vi "devices.vi"(8 "error in (no error)":errorcluster, 11 "reference in":refnum<class "Project Panels.lvclass">=refnum) -> (0 "error out":errorcluster, 3 "reference out":refnum<class "Project Panels.lvclass">)   [LabVIEW 2015, in "Project Panels.lvclass"]
uses:
  Project Panels.lvclass
  state.ctl
  <vilib>/Utility/miscctls.llb/LVRowAndColumnUnsignedTypeDef.ctl
  SYS/Devices Controller_llb/deviceType.ctl
  <vilib>/Utility/miscctls.llb/LVRowAndColumnTypeDef.ctl
  APP/excelFile_class/fileType.ctl
  SYS/Devices Controller_llb/Devices Controller.lvclass
  SYS/File Controller_llb/File Controller.lvclass
  APP/excelFile_class/excelFile.lvclass
panel:
  out "title":string="Cosmed Asia Pacific - Products in Aussie"
  in  "tables":T1(tab)
  out "K5":string[][](table)=[["705001", "not active", "K4b2", "not active", "not active", "not active", "not active", "not active", "not active", "not active", "not active", "not active", ""], ["803033", "not active", "K4b2", "not active", "not active", "not active", "not active", "not active", "not active", "not active", "not active", "not active", ""], ["804042", "not active", "K4b2", "not active", "not active", "not active", "not active", "not active", "not active", "not active", "not active", "not active", ""], ["804046", "", "K4b2", "Univ. of Queensland", "St Lucia, Brisbane", "Gary Wilson", "seant@hms.uq.edu.au", "Bellamby", "sep-06", "Italy", "sep-07", "not active", ""], ["804047", "not active", "K4b2", "not active", "not active", "not active", "not active", "not active", "not active", "not active", "not active", "not active", ""], ["9806059", "6.2", "K4b2", "not active", "not active", "not active", "not active", "not active", "not active", "not active", "not active", "not active", ""], ["9806062", "5.1", "K4b2", "Queensland Academy of Sport", "Sunnybank", "Mark Andrews", "mark.andrews@srq.qld.com.au", "Nahtan, GC", "june 2013 in italy for CO2 refurbish", "Italy service", "jun-14", "", ""], ["9807077", "6.0a", "K4b2", "Uni of Canterbury", "Uni of Canterbury", "Gavin Blackwell", "gavin.blackwell@canterbury.ac.nz", "Christchurch", "feb-13", "fede", "feb-14", "", ""], ["9810080", "", "K4b2", "Royal Children's Hospital", "Herston", "Teresa Phillips", "Teresa_Phillips@health.qld.gov.au", "Herston", "jun-06", "Italy", "jun-07", "9/17/2013", ""], ["9903123", "7.2", "K4b2", "Uni of Adelaide", "Uni of Adelaide", "David Bentley", "david.bentley@adelaide.edu.au", "Adelaide", "dic-12", "Serv Italy +valve", "dic-13", "", ""], ["9912206", "7.3", "K4b2", "Uni of Canterbury", "Uni of Canterbury", "Gavin Blackwell", "gavin.blackwell@canterbury.ac.nz", "Christchurch", "feb-13", "fede", "feb-14", "", ""], ["200104325", "8", "K4b2", "Uni of South Australia", "Sansom Institute", "Michelle N. McDonnell", "", "Adelaide", "nov-11", "fede", "dic-12", "9/9/2013", ""], ["200201385", "9.1b", "K4b2", "University of Sydney", "Lidcombe Campus", "Hui Yin Ler  (PhD)", "", "Sydney", "oct-11", "fede", "oct-12", "9/9/2013", ""], ["200205419", "8.0", "K4b2", "University of Sydney", "Liverpool hospital", "Leanne Hassett", "leanne.hassett@sydney.edu.au", "Sydney", "nov-11", "fede", "nov-12", "Not Using in this moment", ""], ["200205423", "9.1b", "K4b2", "University of Sydney", "Lidcombe Campus", "Martin Thomson", "", "Sydney", "feb-10", "italy", "feb-11", "9/9/2013", ""], ["200205424", "7.3", "K4b2", "University of Sydney", "Lidcombe Campus", "Martin Thomson", "", "Sydney", "sep-08", "Italy", "sep-09", "9/10/2013", ""], ["200404607", "", "K4b2", "The Sydney Children's Hospital Network", "Westmead", "Leanne Purcell", "leanne.purcell@health.nsw.gov.au", "Westmead", "nov-08", "italy", "nov-09", "9/17/2013", "Yes, but waiting the start of the testing"], ["200512701", "8.0b", "K4b2", "James Cook Uni", "James Cook Uni", "Anthony Leight", "Anthony.Leicht@jcu.edu.au", "Townsville", "jan-13", "", "jan-14", "", ""], ["200601705", "", "K4b2", "Latrobe University", "Bundoora (Melb)", "Paul Moon", "P.Moon@latrobe.edu.au", "Melbourne", "jan-08", "Italy", "jan-09", "9/17/2013", ""], ["200607745", "", "K4b2", "QUT Brisbane", "Kelvin Grove", "Pei Cher", "pei.cher@qut.edu.au", "BBN", "may-13", "fede", "may-14", "", ""], ["200710813", "", "K4b2", "Victoria Uni", "", "Jessica Meilak", "jessica.meilak@vu.edu.au", "Melb", "jan-12", "Brad", "jan-14", "15/01/14", ""], ["200907909", "9.1b", "K4b2", "Uni of New South Wales", "Uni of New South Wales", "Stephen Redmond", "s.redmond@unsw.edu.au", "Sydney", "sep-12", "fede", "sep-13", "9/17/2013", ""], ["200909916", "", "K4b2", "Uni of Canterbury", "Uni of Canterbury", "Gavin Blackwell", "gavin.blackwell@canterbury.ac.nz", "Christchurch", "feb-13", "fede", "feb-14", "", ""], ["201007964", "", "K4b2", "University of Canberra", "Canberra", "Ben Rattray", "ben.rattray@canberra.edu.au", "Canberra", "mar-12", "", "mar-13", "9/17/2013", ""], ["201009980", "9.1b", "K4b2", "Uni of Technology Sydney", "UTS City Campus", "Steven Su", "steven.su@eng.uts.edu.au", "Sydney", "oct-12", "Medtel (also Lee Valve)", "oct-13", "9/17/2013", ""], ["2011121063", "", "K4b2", "Victoria Uni", "", "Jessica Meilak", "jessica.meilak@vu.edu.au", "Melb", "jan-12", "Brad", "jan-14", "", ""], ["2011121064", "", "K4b2", "Victoria Uni", "", "Jessica Meilak", "jessica.meilak@vu.edu.au", "Melb", "jan-12", "Brad", "jan-14", "", ""], ["2012021076", "", "K4b2", "Demo Unit", "Demo Unit", "TBD", "", "TBD", "sep-13", "Manu-AUS", "sep-14", "", ""], ["2012021080", "", "K4b2", "Massey Univ.", "Wellington", "Brandon Woolley", "B.Woolley@massey.ac.nz", "Wellington", "nov-13", "Manu-AUS", "nov-14", "", ""], ["2012061109", "", "K4b2", "Griffith University Gold Coast Campus", "Gold Coast", "Anna Boehm", "a.boehm@griffith.edu.au", "Gold Coast", "jul-13", "fede", "jul-14", "", ""], ["2012061115", "10.0d", "K4b2", "University of Newcastle", "Callaghan", "Robin Callister", "Robin.Callister@newcastle.edu.au", "Ourimbah", "nov-13", "Manu-AUS", "nov-14", "", ""], ["2012111144", "10.0d", "K4b2", "University of Newcastle", "Callaghan", "Robin Callister", "Robin.Callister@newcastle.edu.au", "Ourimbah", "nov-13", "Manu-AUS", "nov-14", "", ""], ["2012111148", "", "K4b2", "University of Western Sydney", "PENRITH", "Tara Hamilton", "t.hamilton@uws.edu.au", "PENRITH", "dec-13", "Manu-AUS", "dec-14", "", ""], ["2013011158", "10.0d", "K4b2", "University of the Sunshine Coast", "Maroochydore DC", "Ava Kerr", "akerr@usc.edu.au", "Sippy Downs", "may-13", "new", "may-14", "", ""], ["2013031168", "10.0d", "K4b2", "Australian Catholic University", "Sydney", "Phillip Chapman", "Phillip.Chapman@acu.edu.au", "Sydney", "apr-13", "new", "apr-14", "", ""], ["Prova", "", "Prova", "", "", "", "", "", "", "", "", "", ""]]
  out "k4b2":string[][](table)=[["705001", "not active", "K4b2", "not active", "not active", "not active", "not active", "not active", "not active", "not active", "not active", "not active", ""], ["803033", "not active", "K4b2", "not active", "not active", "not active", "not active", "not active", "not active", "not active", "not active", "not active", ""], ["804042", "not active", "K4b2", "not active", "not active", "not active", "not active", "not active", "not active", "not active", "not active", "not active", ""], ["804046", "", "K4b2", "Univ. of Queensland", "St Lucia, Brisbane", "Gary Wilson", "seant@hms.uq.edu.au", "Bellamby", "sep-06", "Italy", "sep-07", "not active", ""], ["804047", "not active", "K4b2", "not active", "not active", "not active", "not active", "not active", "not active", "not active", "not active", "not active", ""], ["9806059", "6.2", "K4b2", "not active", "not active", "not active", "not active", "not active", "not active", "not active", "not active", "not active", ""], ["9806062", "5.1", "K4b2", "Queensland Academy of Sport", "Sunnybank", "Mark Andrews", "mark.andrews@srq.qld.com.au", "Nahtan, GC", "june 2013 in italy for CO2 refurbish", "Italy service", "jun-14", "", ""], ["9807077", "6.0a", "K4b2", "Uni of Canterbury", "Uni of Canterbury", "Gavin Blackwell", "gavin.blackwell@canterbury.ac.nz", "Christchurch", "feb-13", "fede", "feb-14", "", ""], ["9810080", "", "K4b2", "Royal Children's Hospital", "Herston", "Teresa Phillips", "Teresa_Phillips@health.qld.gov.au", "Herston", "jun-06", "Italy", "jun-07", "9/17/2013", ""], ["9903123", "7.2", "K4b2", "Uni of Adelaide", "Uni of Adelaide", "David Bentley", "david.bentley@adelaide.edu.au", "Adelaide", "dic-12", "Serv Italy +valve", "dic-13", "", ""], ["9912206", "7.3", "K4b2", "Uni of Canterbury", "Uni of Canterbury", "Gavin Blackwell", "gavin.blackwell@canterbury.ac.nz", "Christchurch", "feb-13", "fede", "feb-14", "", ""], ["200104325", "8", "K4b2", "Uni of South Australia", "Sansom Institute", "Michelle N. McDonnell", "", "Adelaide", "nov-11", "fede", "dic-12", "9/9/2013", ""], ["200201385", "9.1b", "K4b2", "University of Sydney", "Lidcombe Campus", "Hui Yin Ler  (PhD)", "", "Sydney", "oct-11", "fede", "oct-12", "9/9/2013", ""], ["200205419", "8.0", "K4b2", "University of Sydney", "Liverpool hospital", "Leanne Hassett", "leanne.hassett@sydney.edu.au", "Sydney", "nov-11", "fede", "nov-12", "Not Using in this moment", ""], ["200205423", "9.1b", "K4b2", "University of Sydney", "Lidcombe Campus", "Martin Thomson", "", "Sydney", "feb-10", "italy", "feb-11", "9/9/2013", ""], ["200205424", "7.3", "K4b2", "University of Sydney", "Lidcombe Campus", "Martin Thomson", "", "Sydney", "sep-08", "Italy", "sep-09", "9/10/2013", ""], ["200404607", "", "K4b2", "The Sydney Children's Hospital Network", "Westmead", "Leanne Purcell", "leanne.purcell@health.nsw.gov.au", "Westmead", "nov-08", "italy", "nov-09", "9/17/2013", "Yes, but waiting the start of the testing"], ["200512701", "8.0b", "K4b2", "James Cook Uni", "James Cook Uni", "Anthony Leight", "Anthony.Leicht@jcu.edu.au", "Townsville", "jan-13", "", "jan-14", "", ""], ["200601705", "", "K4b2", "Latrobe University", "Bundoora (Melb)", "Paul Moon", "P.Moon@latrobe.edu.au", "Melbourne", "jan-08", "Italy", "jan-09", "9/17/2013", ""], ["200607745", "", "K4b2", "QUT Brisbane", "Kelvin Grove", "Pei Cher", "pei.cher@qut.edu.au", "BBN", "may-13", "fede", "may-14", "", ""], ["200710813", "", "K4b2", "Victoria Uni", "", "Jessica Meilak", "jessica.meilak@vu.edu.au", "Melb", "jan-12", "Brad", "jan-14", "15/01/14", ""], ["200907909", "9.1b", "K4b2", "Uni of New South Wales", "Uni of New South Wales", "Stephen Redmond", "s.redmond@unsw.edu.au", "Sydney", "sep-12", "fede", "sep-13", "9/17/2013", ""], ["200909916", "", "K4b2", "Uni of Canterbury", "Uni of Canterbury", "Gavin Blackwell", "gavin.blackwell@canterbury.ac.nz", "Christchurch", "feb-13", "fede", "feb-14", "", ""], ["201007964", "", "K4b2", "University of Canberra", "Canberra", "Ben Rattray", "ben.rattray@canberra.edu.au", "Canberra", "mar-12", "", "mar-13", "9/17/2013", ""], ["201009980", "9.1b", "K4b2", "Uni of Technology Sydney", "UTS City Campus", "Steven Su", "steven.su@eng.uts.edu.au", "Sydney", "oct-12", "Medtel (also Lee Valve)", "oct-13", "9/17/2013", ""], ["2011121063", "", "K4b2", "Victoria Uni", "", "Jessica Meilak", "jessica.meilak@vu.edu.au", "Melb", "jan-12", "Brad", "jan-14", "", ""], ["2011121064", "", "K4b2", "Victoria Uni", "", "Jessica Meilak", "jessica.meilak@vu.edu.au", "Melb", "jan-12", "Brad", "jan-14", "", ""], ["2012021076", "", "K4b2", "Demo Unit", "Demo Unit", "TBD", "", "TBD", "sep-13", "Manu-AUS", "sep-14", "", ""], ["2012021080", "", "K4b2", "Massey Univ.", "Wellington", "Brandon Woolley", "B.Woolley@massey.ac.nz", "Wellington", "nov-13", "Manu-AUS", "nov-14", "", ""], ["2012061109", "", "K4b2", "Griffith University Gold Coast Campus", "Gold Coast", "Anna Boehm", "a.boehm@griffith.edu.au", "Gold Coast", "jul-13", "fede", "jul-14", "", ""], ["2012061115", "10.0d", "K4b2", "University of Newcastle", "Callaghan", "Robin Callister", "Robin.Callister@newcastle.edu.au", "Ourimbah", "nov-13", "Manu-AUS", "nov-14", "", ""], ["2012111144", "10.0d", "K4b2", "University of Newcastle", "Callaghan", "Robin Callister", "Robin.Callister@newcastle.edu.au", "Ourimbah", "nov-13", "Manu-AUS", "nov-14", "", ""], ["2012111148", "", "K4b2", "University of Western Sydney", "PENRITH", "Tara Hamilton", "t.hamilton@uws.edu.au", "PENRITH", "dec-13", "Manu-AUS", "dec-14", "", ""], ["2013011158", "10.0d", "K4b2", "University of the Sunshine Coast", "Maroochydore DC", "Ava Kerr", "akerr@usc.edu.au", "Sippy Downs", "may-13", "new", "may-14", "", ""], ["2013031168", "10.0d", "K4b2", "Australian Catholic University", "Sydney", "Phillip Chapman", "Phillip.Chapman@acu.edu.au", "Sydney", "apr-13", "new", "apr-14", "", ""], ["Prova", "", "Prova", "", "", "", "", "", "", "", "", "", ""]]
  out "fitmate":string[][](table)=[["2005090013", "2.2", "Fitmate Pro", "Wesley Weight Management", "Milton", "Liz Ernst", "eernst@lifeshape.com.au", "Milton", "27/09", ""], ["2006020058", "1", "Fitmate WM", "Toombul Medical Centre", "Spring Hill", "Zoe Glover", "toombulmc@gmail.com", "Spring Hill", "27/09", ""], ["2006020059", "1", "Fitmate WM", "RMIT Univ.", "Melbourne", "George Lenon", "george.lenon@rmit.edu.au", "Melbourne", "27/09", ""], ["2006020060", "1", "Fitmate WM", "Logan Hospital", "Meadowbrook", "??", "??", "Meadowbrook", "", ""], ["2006020061", "1.6", "Fitmate WM", "Biomedex (Aust) Pty Ltd", "Woonona", "Biomedex (Aust) Pty Ltd", "??", "Woonona", "", ""], ["2006020077", "1", "Fitmate Pro", "Wesley Weight Management", "Southport", "Sally Jordan", "SJordan@weshealth.com.au", "Southport", "27/09 mail come back / no problem", ""], ["2006020078", "1", "Fitmate Pro", "Life4Ever Pty Ltd", "Arundel", "Michael Tait", "mail@drmichaeltait.com", "Arundel", "27/09 mail come back", ""], ["2006030062", "2.2", "Fitmate WM", "Biomedex (Aust) Pty Ltd", "Woonona", "Biomedex (Aust) Pty Ltd", "??", "Woonona", "", ""], ["2006030083", "2", "Fitmate Pro", "Australian College of Physical Education", "Olympic Park Sydney", "Sven Rees", "srees@acpe.edu.au", "Olympic Park Sydney", "30/09", ""], ["2006030084", "2.3", "Fitmate Pro", "Monash Univ. The Alfred Centre", "Frankston", "Tim Wallace", "tim.wallace@monash.edu", "Frankston", "Case Opned for Macro error", ""], ["2006030085", "2.2", "Fitmate Pro", "Southside Exercise Therapy", "Gymea", "Luke Delvecchio", "southsidepty@optusnet.com.au", "Gymea", "30/09", ""], ["2006060076", "1.1", "Fitmate WM", "Edith Cowan Univ.", "Joondalup", "Amanda Devine", "a.devine@ecu.edu.au", "Joondalup", "30/09", ""], ["2006060078", "1.1", "Fitmate WM", "Edith Cowan Univ.", "Joondalup", "Amanda Devine", "a.devine@ecu.edu.au", "Joondalup", "30/09", ""], ["2006060080", "2.3", "Fitmate WM", "WESLEY Corporate Health", "Brisbane", "Liz Ernst", "eernst@lifeshape.com.au", "Brisbane", "27/09", ""], ["2006080185", "1.1", "Fitmate Pro", "Edith Cowan Univ.", "Joondalup", "Doreen Mackie", "DMackie@hotmail.com", "Joondalup", "Waiting for details from email (n.vrdoljak@ecu.edu.au   )", ""], ["2006080186", "1.1", "Fitmate Pro", "Neocardia PTY LTD", "Noosaville", "Neavison", "Neavison@hotmail.com", "Noosaville", "30/09", ""], ["2006080187", "1.1", "Fitmate Pro", "Kams Health and Fitness", "Armidale", "Kamahl Barhoush", "info@kams.com.au", "Armidale", "doesn't answer/call again", ""], ["2006080188", "1.1", "Fitmate Pro", "Edith Cowan Univ.", "Joondalup", "Doreen Mackie", "DMackie@hotmail.com", "Joondalup", "Waiting for details from email (n.vrdoljak@ecu.edu.au   )", ""], ["2006080189", "1.1", "Fitmate Pro", "Get Back On Track", "Victoria", "Lisa Ham", "LisaH@bigpond.com.au", "Victoria", "doesn't answer/call again", ""], ["2006080190", "1.1", "Fitmate Pro", "Edith Cowan Univ.", "Joondalup", "Doreen Mackie", "DMackie@hotmail.com", "Joondalup", "Waiting for details from email (n.vrdoljak@ecu.edu.au   )", ""], ["2006080191", "1.1", "Fitmate Pro", "One Life", "PADDINGTON", "Justin Lang", "admin@onelifeliveit.net.au", "PADDINGTON", "01/10", "NOT ACTIVE"], ["2007030363", "1.1", "Fitmate Pro", "X-Fitness Systems Ltd", "Auckland,", "Scott Tibbutt", "scott@xfitness.co.nz", "Auckland,", "30/09", ""], ["2007030372", "1.1", "Fitmate Pro", "Edith Cowan Univ.", "Joondalup", "Doreen Mackie", "DMackie@hotmail.com", "Joondalup", "Waiting for details from email (n.vrdoljak@ecu.edu.au   )", ""], ["2007030373", "1.1", "Fitmate Pro", "Edith Cowan Univ.", "Joondalup", "Doreen Mackie", "DMackie@hotmail.com", "Joondalup", "Waiting for details from email (n.vrdoljak@ecu.edu.au   )", ""], ["2007030375", "1.1", "Fitmate Pro", "Vision Health and Fitness", "Toowoomba", "Troy Taylor", "troy@visionhealth.com.au", "Toowoomba", "30/09", ""], ["2007050155", "2", "Fitmate WM", "Fitness Fusion", "Ohope", "Erin Baker", "paul@fitnessfusion.co.nz", "Ohope", "30/09", ""], ["2007050156", "1.1", "Fitmate WM", "X-Fitness Systems Ltd", "Auckland,", "X-Fitness Systems Ltd", "jeremyu@uhl.co.nz", "Auckland,", "30/09", ""], ["2007050157", "2.2", "Fitmate WM", "Wesley Weight Management", "Milton", "Liz Ernst", "eernst@lifeshape.com.au", "Milton", "27/09", ""], ["2007050158", "2.2", "Fitmate WM", "WESLEY Corporate Health", "Brisbane", "Liz Ernst", "eernst@lifeshape.com.au", "Brisbane", "27/09", ""], ["2007050159", "1.1", "Fitmate WM", "Wesley Weight Management", "Rockhampton", "Simon Fawssett", "sfawssett@weshealth.com.au", "Rockhampton", "no problem", ""], ["2007050160", "2.2", "Fitmate WM", "WESLEY Corporate Health", "Brisbane", "Liz Ernst", "eernst@lifeshape.com.au", "Brisbane", "27/09", ""], ["2007050161", "1.1", "Fitmate WM", "Pyrmont Health & Fitness Club", "Pyrmont", "Antoine Poulter", "??", "Pyrmont", "", ""], ["2007050376", "1.1", "Fitmate Pro", "Edith Cowan Univ.", "Joondalup", "Doreen Mackie", "DMackie@hotmail.com", "Joondalup", "Waiting for details from email (n.vrdoljak@ecu.edu.au   )", ""], ["2007050377", "1.1", "Fitmate Pro", "Elgin Street Medical Centre", "Carlton", "Daniel Cobb", "dcobb@live.com.au", "Carlton", "30/09", ""], ["2007050378", "1.1", "Fitmate Pro", "Pyrmont Health & Fitness Club", "Pyrmont", "Justine Justine", "??", "Pyrmont", "", ""], ["2007050379", "1.6", "Fitmate Pro", "HERT", "Millers Point", "Mark Newton", "mark@hert.com.au", "Millers Point", "30/09", ""], ["2007050380", "1.1", "Fitmate Pro", "Edith Cowan Univ.", "Joondalup", "Doreen Mackie", "DMackie@hotmail.com", "Joondalup", "Waiting for details from email (n.vrdoljak@ecu.edu.au   )", ""], ["2007050381", "1.6", "Fitmate Pro", "Fitness Development Australia", "Sydney", "Fitness Development Australia", "zarko_mikulic@hotmail.com", "Sydney", "30/09", ""], ["2007050388", "1.1", "Fitmate Pro", "ULO Pty Ltd", "Roebourne Court", "Adam Brown", "adam@ulo.com.au", "Daisy Hill", "30/09", ""], ["2007050395", "1.6", "Fitmate Pro", "Biomedex (Aust) Pty Ltd", "Woonona", "Biomedex (Aust) Pty Ltd", "??", "Woonona", "", ""], ["2007050404", "1.1", "Fitmate Pro", "Biomedex (Aust) Pty Ltd", "Woonona", "Biomedex (Aust) Pty Ltd", "??", "Woonona", "", ""], ["2007060413", "2", "Fitmate Pro", "Biomedex (Aust) Pty Ltd", "Woonona", "Biomedex (Aust) Pty Ltd", "??", "Woonona", "", ""], ["2007060415", "1.1", "Fitmate Pro", "Mater Childrens Hospital", "South Brisbane", "Gary Leong", "gary.leong@mater.org.au", "South Brisbane", "1/10/2013", ""], ["2007060417", "1.1", "Fitmate Pro", "Ray Kelly Fitness", "Blacktown", "Ray Kelly", "maxvel01@hotmail.com", "Blacktown", "30/09", ""], ["2007100277", "2.2", "Fitmate WM", "Biomedex (Aust) Pty Ltd", "Woonona", "Biomedex (Aust) Pty Ltd", "??", "Woonona", "", ""], ["2007100278", "1.1", "Fitmate WM", "Tone Up Weight Loss", "Campbelltown", "Christopher Satara", "scott@swphysio.com.au'", "Campbelltown", "08/10", ""], ["2007100279", "1.6", "Fitmate WM", "Biomedex (Aust) Pty Ltd", "Woonona", "Biomedex (Aust) Pty Ltd", "??", "Woonona", "", ""], ["2007100281", "2.2", "Fitmate WM", "Biomedex (Aust) Pty Ltd", "Woonona", "Biomedex (Aust) Pty Ltd", "??", "Woonona", "", ""], ["2007100282", "2.2", "Fitmate WM", "Biomedex (Aust) Pty Ltd", "Woonona", "Biomedex (Aust) Pty Ltd", "??", "Woonona", "", ""], ["2007100484", "2.3", "Fitmate Pro", "Univ. of Auckland", "Auckland", "Grant Mawston", "", "Auckland", "", ""], ["2008010568", "2.3", "Fitmate Pro", "Australian College of", "Olympic Park Sydney", "Sven Rees", "srees@acpe.edu.au", "Olympic Park Sydney", "30/09", ""], ["2008010576", "2.2", "Fitmate Pro", "Body Dynamics Illawarra", "Bulli", "Alan Wilkie", "alan@bodydynamics.com.au", "Bulli", "01/10", ""], ["2008010578", "2.2", "Fitmate Pro", "Cardiofirst Pty Ltd.", "Frenchs Forest", "Camilla", "reports@cardiofirst.com.au", "Frenchs Forest", "", ""], ["2008010579", "2.2", "Fitmate Pro", "Biomedex (Aust) Pty Ltd", "Woonona", "Biomedex (Aust) Pty Ltd", "??", "Woonona", "", ""], ["2008010585", "1.1", "Fitmate Pro", "Biomedex (Aust) Pty Ltd", "Woonona", "Biomedex (Aust) Pty Ltd", "??", "Woonona", "", ""], ["2008030035", "1.6", "Fitmate MED", "Biomedex (Aust) Pty Ltd", "Woonona", "Biomedex (Aust) Pty Ltd", "??", "Woonona", "", ""], ["2008030037", "2", "Fitmate MED", "Biomedex (Aust) Pty Ltd", "Woonona", "Biomedex (Aust) Pty Ltd", "??", "Woonona", "", ""], ["2008040639", "1.5", "Fitmate Pro", "", "Wellington", "Stefan Darrall", "stefan.darrall@xtra.co.nz", "Wellington", "01/10", ""], ["2008040645", "2,2", "Fitmate Pro", "FEDERICO ZANELLA", "Narrabeen", "Federico Zanella", "", "Narrabeen", "", ""], ["2008090067", "2", "Fitmate MED", "Biomedex Pty Ltd.", "Bellambi", "Biomedex Pty Ltd.", "??", "Bellambi", "", ""], ["2008090071", "2", "Fitmate MED", "Logan City Council", "Logan Central", "Campbell MacGregor (not work there anymore)", "council@logan.qld.gov.au", "Logan Central", "08/10 request info sent", ""], ["2008090073", "1.6", "Fitmate MED", "Biomedex (Aust) Pty Ltd", "Woonona", "Biomedex (Aust) Pty Ltd", "??", "Woonona", "", ""], ["2008090075", "1.6", "Fitmate MED", "Enriched Health and Fizzsport Physiotherapy", "Port Macquarie", "Simon Turnball", "simon.turnbull@enrichedhealth.com.au", "Port Macquarie", "01/10", ""], ["2008090076", "2", "Fitmate MED", "Biomedex Pty Ltd.", "Bellambi", "Biomedex Pty Ltd.", "??", "Bellambi", "", ""], ["2008100402", "1.6", "Fitmate WM", "LSNDS P/L", "Mount Eliza", "Andrew Harland", "lsnds@optusenet.com.au", "Mount Eliza", "", ""], ["2008100403", "2.2", "Fitmate WM", "Monash Univ. The Alfred Centre", "Melbourne", "Emma Ridley", "emma.ridley@monash.edu", "Melbourne", "01/10", ""], ["2008100404", "1.6", "Fitmate WM", "The Prince Charles Hospital", "Brisbane", "Renee Rogers", "", "Brisbane", "", ""], ["2008100405", "2.2", "Fitmate WM", "Monash Univ. The Alfred Centre", "Melbourne", "Emma Ridley", "emma.ridley@monash.edu", "Melbourne", "01/10", ""], ["2008100408", "1.6", "Fitmate WM", "Univ. of Newcastle (AUSTRALIA)", "Tamworth", "Leanne Brown", "leanne.brown@newcastle.edu.au", "Tamworth", "01/10", ""], ["2009070009", "1,6", "Fitmate Pro", "Ray Kelly Fitness", "Blacktown", "Ray Kelly", "maxvel01@hotmail.com", "Blacktown", "30/09", ""], ["2010011057", "2", "Fitmate Pro", "Swift Sports Performance Equip", "Lismore", "Mark Fisher", "mark@spe.com.au", "Lismore", "01/10", ""], ["2010021097", "2", "Fitmate Pro", "ASCENCIA Pty. Limited", "Notting Hill", "Michael Panagopoulos", "michael@ascencia.com.au", "Notting Hill", "", ""], ["2010021098", "2", "Fitmate Pro", "Melbourne Sports & Allied Health Clinic", "Essendon North", "Simon Sostaric", "simon@msahc.com.au", "Essendon North", "01/10", ""], ["2010041123", "2", "Fitmate Pro", "Pymble Ladies College", "Pymble", "Thomas Kindred", "tkindred@pymblelc.nsw.edu.au", "Pymble", "01/10", ""], ["2010041133", "2", "Fitmate Pro", "New Zealand Institute of Sport", "Wellington", "Tony Rogers", "tony.r@nzis.co.nz", "Wellington", "info da fede", ""], ["2010091200", "2", "Fitmate Pro", "Univ. of Western Sydney", "Sydney", "Andrew Webber", "a.webber@uws.edu.au / a.boros@uws.edu.au", "Sydney", "01/10", ""], ["2010091208", "2.2", "Fitmate Pro", "AusFitness Test", "Burleigh Heads", "Daniel Mckenzie", "dan@ausfitnesstest.com", "Burleigh Heads", "01/10", ""], ["2010111079", "2", "Fitmate MED", "Xceler8", "Wagga", "Kerry Podmore", "Kerry-xceler8@bigpond.com", "Wagga", "01/10", ""], ["2010121080", "2", "Fitmate MED", "", "Toormina, Boambee", "Chris Cherry", "", "Toormina, Boambee", "", ""], ["2010121084", "2", "Fitmate MED", "Victoria University", "St.ALbans", "Christos Stathis", "christos.stathis@vu.edu.au", "St.ALbans", "01/10", ""], ["2010121085", "2", "Fitmate MED", "Victoria University", "St.ALbans", "Christos Stathis", "christos.stathis@vu.edu.au", "St.ALbans", "01/10", ""], ["2010121088", "2", "Fitmate MED", "", "Melbourne Nth.", "T. Goh", "??", "Melbourne Nth.", "", ""], ["2010121250", "2.2", "Fitmate Pro", "Otago Polytechnic", "Dunedin", "Hayden Croft", "Hayden.Croft@op.ac.nz", "Dunedin", "01/10", ""], ["2011021095", "2", "Fitmate MED", "CHM Management", "South Melbourne", "Kirsty Lerm", "klerm@chm.com.au", "South Melbourne", "01/10", ""], ["2011041238", "2.2", "Fitmate WM", "University of the Sunshine Coast", "Sippy Downs", "Gary Slater", "gslater@usc.edu.au", "Maroochydore DC", "01/10", "accepted 04/10"], ["2011061360", "2.2", "Fitmate Pro", "Sports Orthopaedic and Rehabilitation", "Sydney", "Peter McDonald", "pmcdfitness@gmail.com.au'", "Sydney", "", ""], ["2011061363", "2.2", "Fitmate Pro", "Sports Orthopaedic and Rehabilitation", "Sydney", "Peter McDonald", "pmcdfitness@gmail.com.au'", "Sydney", "", ""], ["2011071270", "2.2", "Fitmate WM", "University of Otago", "Dunedin", "Gavin Hendry", "gavin.hendry@otago.ac.nz", "Dunedin", "01/10", ""], ["2011111148", "2", "Fitmate MED", "JLM Accutek Health", "Homebush", "Lorrence(Lorenzo) Platania", "??", "Homebush", "", ""], ["2011111155", "2", "Fitmate MED", "JLM Accutek Health", "Homebush", "Lorrence(Lorenzo) Platania", "??", "Homebush", "", ""], ["2011121441", "2.2", "Fitmate Pro", "The Scots College", "Bellevue Hill", "Tenzing Tsewang", "t.tsewang@tsc.nsw.edu.au", "Bellevue Hill", "01/10", ""], ["2011121443", "2.2", "Fitmate Pro", "Sydney Sports & Exercise", "Sydney Olympic Park", "Dean McNamara", "", "Sydney Olympic Park", "", ""], ["2012031327", "2.2", "Fitmate WM", "Univ. of Adelaide", "Adelaide", "Univ. of Adelaide", "", "Adelaide", "", ""], ["2012050009", "2,3", "Fitmate GS", "Belconnen Specialist Center", "Bruce-Canberra", "Mariame Iraki", "", "Bruce-Canberra", "", ""], ["2012061551", "2.2", "Fitmate Pro", "The Scots College", "Bellevue Hill", "Tenzing Tsewang", "t.tsewang@tsc.nsw.edu.au", "Bellevue Hill", "01/10", ""], ["2012061552", "2.2", "Fitmate Pro", "The Scots College", "Bellevue Hill", "Tenzing Tsewang", "t.tsewang@tsc.nsw.edu.au", "Bellevue Hill", "01/10", ""], ["2012061554", "2.2", "Fitmate Pro", "The Scots College", "Bellevue Hill", "Tenzing Tsewang", "t.tsewang@tsc.nsw.edu.au", "Bellevue Hill", "01/10", ""], ["2012091028", "2,3", "Fitmate GS", "The University of Newcastle (AUS)", "Callaghan", "Anna Bukey", "Anna.Bukey@newcastle.edu.au", "Callaghan", "01/10", ""], ["2012101617", "2.3", "Fitmate Pro", "FEDERICO ZANELLA", "Narrabeen", "Federico Zanella", "", "Narrabeen", "", ""], ["2012101619", "2.3", "Fitmate Pro", "Adelaide Exercise Physiology (AEP)", "", "Reuben Vanderzalm", "reuben@aep.net.au", "", "01/10", ""], ["2012111654", "2.2", "Fitmate Pro", "Vascular Ultrasound Partners Pty Ltd", "Adelaide", "Jim Gotting", "emac2403@gmail.com", "Adelaide", "01/10", ""], ["2013011031", "2,3", "Fitmate GS", "FEDERICO ZANELLA", "Narrabeen", "Federico Zanella", "", "Narrabeen", "", ""], ["2013021388", "2.2", "Fitmate WM", "Monash Univ. The Alfred Centre", "Melbourne", "Emma Ridley", "emma.ridley@monash.edu", "Melbourne", "01/10", ""], ["2013041734", "2.2", "Fitmate Pro", "SA Ambulance", "Eastwood", "Adam Zerner", "adam.zerner@health.sa.gov.au", "Eastwood", "01/10", ""], ["2013061753", "2.2", "Fitmate Pro", "James Cook University", "Douglas", "Anthony Leight", "Anthony.Leicht@jcu.edu.au", "Townsville", "01/10", ""], ["20050800003", "1.6", "Fitmate Pro", "Biomedex (Aust) Pty Ltd", "Woonona", "Biomedex (Aust) Pty Ltd", "??", "Woonona", "", ""]]
  out "RMR":string[][](table)=[["2009010042", "", "RMR + ICU", "Monash Univ. The Alfred Centre", "Melbourne", "Emma Ridley", "Emma.Ridley@med.monash.edu.au", "Melbourne", "", ""], ["2010020172", "", "RMR + ICU", "Prince Charles Hospital", "Brisbane", "Vanessa King", "Vanessa_King@health.qld.gov.au", "Brisbane", "", ""], ["2010080174", "", "RMR + ICU", "Monash Univ. The Alfred Centre", "Melbourne", "Emma Ridley", "Emma.Ridley@med.monash.edu.au", "Melbourne", "", ""], ["2010110180", "", "RMR + ICU", "Monash Univ. The Alfred Centre", "Melbourne", "Emma Ridley", "Emma.Ridley@med.monash.edu.au", "Melbourne", "", ""], ["2010110181", "", "RMR + ICU", "Gold Coast Hospital and Robina", "Southport", "Alan Spencer", "alan_spencer@healthqld.gov.au", "Southport", "", ""], ["2011050212", "", "RMR + ICU", "John Hunter Hospital", "New Lambton Heights", "Justin Singleton", "justin.singleton@hnehealth.nsw.gov.au", "New Lambton Heights", "", ""], ["2011110238", "", "RMR", "Royal Prince Alfred Hospital", "Camperdown", "Joanne Heyman", "joanne.heyman@sswahs.nsw.gov.au", "Camperdown", "", ""], ["2012110294", "", "RMR", "University of the Sunshine Coast", "Maroochydore DC", "Gary Slater", "gslater@usc.edu.au", "Maroochydore DC", "", ""], ["2013020316", "", "RMR + ICU", "Royal Perth Hospital", "Perth", "Wayne Epton", "wayne.epton@health.wa.gov.au", "Perth", "", ""], ["2013050335", "", "RMR + ICU", "Gold Coast Hospital and Robina", "Southport", "Alan Spencer", "alan_spencer@healthqld.gov.au", "Southport", "", ""], ["2013050332", "", "RMR", "Auckland City Hospital", "Auckland", "Shay McGuinness", "", "Auckland", "", ""], ["2013050330", "", "RMR + ICU", "University of Queensland", "Herston", "Alexia Murphy", "alexia.murphy@uq.edu.au", "Herston", "", ""]]
  out "CPET":string[][](table)=[["9807035", "5", "Quark b2", "The Royal Melbourne Institute of Technology - RMIT", "Bundoora", "", "", "", "", ""], ["9901046", "", "Quark b2", "Biomedex", "", "", "", "", "", ""], ["9905053", "5.1a", "Quark b2", "Baker Medical Research Institute", "", "", "", "", "", ""], ["200601281", "", "Quark b2", "Ultra Thoroughbred Racing Pty. Ltb", "Green Iris", "Rod Cedaro", "rod.cedaro@gmail.com", "Rod Cedaro", "", ""], ["2007060003", "", "Quark CPET", "Liverpool Hospital", "Liverpool", "Mark Newman", "Mark.Newman@sswahs.nsw.gov.au", "Liverpool", "", ""], ["2008030037", "10.0d", "Quark CPET", "University Otago", "Dunedin", "Nigel Barrett", "nigel.barrett@otago.ac.nz", "Dunedin", "", ""], ["2008030006", "", "Quark PFT/CPET Nutritional", "University Otago", "Dunedin", "Dene Irvine", "dene.irvine@otago.ac.nz", "Dunedin", "", ""], ["2008050039", "9", "Quark CPET", "Victorian Institute of Sport", "Melbourne", "Simon Blundell", "simon.blundell@vis.org.au", "Melbourne", "", ""], ["2008120093", "9.1b", "Quark CPET", "Griffith University Gold Coast Campus", "Gold Coast", "Caroline Young", "caroline.b.young@griffith.edu.au", "Gold Coast", "", ""], ["2009100185", "10.0d", "Quark CPET", "University of Otago", "Dunedin", "Nigel Barrett", "nigel.barrett@otago.ac.nz", "Dunedin", "", ""], ["2010020214", "", "Quark CPET", "Canberra Hospital", "Garran", "Leonard Arnolda", "", "Garran", "", ""], ["2011110397", "10.0d", "Quark CPET", "Univ. of Sydney", "Lidcombe", "Corinne Caillaud", "corinnecalillaud@sidney.edu.au", "Lidcombe", "", ""], ["2011110398", "10.0d", "Quark CPET", "Univ. of Sydney", "Lidcombe", "Corinne Caillaud", "corinnecalillaud@sidney.edu.au", "Lidcombe", "", ""], ["2012020412", "10.0d", "Quark CPET", "University of Otago", "Dunedin", "Nigel Barrett", "nigel.barrett@otago.ac.nz", "Dunedin", "", ""], ["2011120402", "10.0d", "Quark CPET", "The Scots College", "Bellevue Hill", "Tenzing Tsewang", "t.tsewang@tsc.nsw.edu.au", "Bellevue Hill", "", ""], ["2012100477", "10.0d", "Quark CPET", "Victoria University", "Footscray", "Jessica Meilak", "jessica.meilak@vu.edu.au", "Footscray", "", ""], ["2012060085", "10.0d", "Quark CPET", "Victoria University", "Melbourne", "Bradley Gatt", "bradley.gatt@vu.edu.au", "Melbourne", "", ""], ["2012120094", "10.0e", "Quark CPET", "Fede", "DEMO", "DEMO", "DEMO", "DEMO", "", ""], ["2013020524", "", "Quark CPET", "Australian Catholic University - ACU", "Strathfield", "Anoj Poudyal", "anoj.poudyal@acu.edu.au", "Strathfield", "", ""], ["2013060561", "", "Quark CPET", "James Cook University", "Townsville", "Anthony Leight", "Anthony.Leicht@jcu.edu.au", "Douglas", "", ""], ["2013110612", "", "Quark CPET", "Australian Catholic University BBN", "Virginia", "Tim Blackmore", "tim.blackmore@acu.edu.au", "Banyo", "", ""], ["2013120110", "", "Quark CPET", "Australian Catholic University BBN", "Virginia", "Tim Blackmore", "tim.blackmore@acu.edu.au", "Banyo", "", ""]]
  out "BB-PFT":string[][](table)=[["2009010042", "", "RMR + ICU", "Monash Univ. The Alfred Centre", "Melbourne", "Emma Ridley", "Emma.Ridley@med.monash.edu.au", "Melbourne", "", ""], ["2010020172", "", "RMR + ICU", "Prince Charles Hospital", "Brisbane", "Vanessa King", "Vanessa_King@health.qld.gov.au", "Brisbane", "", ""], ["2010080174", "", "RMR + ICU", "Monash Univ. The Alfred Centre", "Melbourne", "Emma Ridley", "Emma.Ridley@med.monash.edu.au", "Melbourne", "", ""], ["2010110180", "", "RMR + ICU", "Monash Univ. The Alfred Centre", "Melbourne", "Emma Ridley", "Emma.Ridley@med.monash.edu.au", "Melbourne", "", ""], ["2010110181", "", "RMR + ICU", "Gold Coast Hospital and Robina", "Southport", "Alan Spencer", "alan_spencer@healthqld.gov.au", "Southport", "", ""], ["2011050212", "", "RMR + ICU", "John Hunter Hospital", "New Lambton Heights", "Justin Singleton", "justin.singleton@hnehealth.nsw.gov.au", "New Lambton Heights", "", ""], ["2011110238", "", "RMR", "Royal Prince Alfred Hospital", "Camperdown", "Joanne Heyman", "joanne.heyman@sswahs.nsw.gov.au", "Camperdown", "", ""], ["2012110294", "", "RMR", "University of the Sunshine Coast", "Maroochydore DC", "Gary Slater", "gslater@usc.edu.au", "Maroochydore DC", "", ""], ["2013020316", "", "RMR + ICU", "Royal Perth Hospital", "Perth", "Wayne Epton", "wayne.epton@health.wa.gov.au", "Perth", "", ""], ["2013050335", "", "RMR + ICU", "Gold Coast Hospital and Robina", "Southport", "Alan Spencer", "alan_spencer@healthqld.gov.au", "Southport", "", ""], ["2013050332", "", "RMR", "Auckland City Hospital", "Auckland", "Shay McGuinness", "", "Auckland", "", ""], ["2013050330", "", "RMR + ICU", "University of Queensland", "Herston", "Alexia Murphy", "alexia.murphy@uq.edu.au", "Herston", "", ""]]
  out "BP":string[][](table)=[["1018", "", "BP GS", "Uni of Adelaide", "Adelaide", "", "", "", "", ""], ["3054", "", "BP DOS", "Uni of Queensland", "Brisbane", "", "", "", "", ""], ["3268", "", "BP DOS W", "Queensland Univ. of Technology", "Kelvin grove", "Rachel Wood", "re.wood@qut.edu.au", "Kelvin grove", "", ""], ["3367", "", "BP W", "Queensland University of Technology", "Kelvin Grove", "Rachel Wood", "re.wood@qut.edu.au", "", "", ""], ["3436", "", "BP W", "Princess Margaret Hospital for Children", "Perth", "David Forbes", "david.forbes@health.wa.gov.au", "Perth", "", ""], ["3529", "5.1.0", "BP GS", "Monash Medical Centre", "Clayton", "Sharon Marks", "sharon@fpds.com.au", "Clayton", "", ""], ["3562", "", "BP GS", "Massey University", "Palmerston North", "Kevin Pedley", "k.c.pedley@massey.ac.nz", "Palmerston North", "", ""], ["3563", "4.2.4", "BP GS", "Bodyology Exercise Science Studio", "Notting Hill", "Andrew Garlick", "andrew@bodyologystudio.com.au", "Notting Hill", "", ""], ["3640", "", "BP GS", "Wesley Research Institute", "Toowong", "Greg Hafner", "ghafner@wesleyresearch.com.au", "Toowong", "", ""], ["3788", "", "BP GS", "Federico", "Federico", "Federico", "", "Federico", "", ""], ["3793", "", "BP GS", "University of the Sunshine Coast", "Maroochydore DC", "Gary Slater", "gslater@usc.edu.au", "Maroochydore DC", "", ""], ["3821", "", "BP GS", "The Scots College", "Bellevue Hill", "Tenzing Tsewang", "t.tsewang@tsc.nsw.edu.au", "Bellevue Hill", "", ""], ["3852", "", "BP GS", "Univ. of Adelaide", "Adelaide", "Univ. of Adelaide", "", "Adelaide", "", ""], ["3868", "5.2.0", "BP GS", "Univ. of Sydney", "Sydney", "Amanda Sainsbury Salis", "amanda.sainsbury-salis@sydney.edu.au", "Sydney", "", ""], ["3930", "", "BP GS", "Paula Serena Pool", "Townsville", "Paula Serena Pool", "", "Townsville", "", ""], ["3947", "", "BP GS", "Paula Serena Pool", "Townsville", "Paula Pool", "", "West End", "", ""], ["3993", "", "BP GS", "Queensland Univ. of Technology", "Kelvin grove", "Nuala Byrne", "n.byrne@qut.edu.au", "Kelvin grove", "", ""], ["4063", "", "BP ST", "Queensland Univ. of Technology", "Kelvin grove", "Rachel Wood", "re.wood@qut.edu.au", "Kelvin grove", "", ""], ["4539", "", "BP EX", "World Gym Ashmore", "Ashmore", "Sarah Friebe", "sarah@worldgymashmore.com.au", "Ashmore", "", ""], ["COSEMD USA 1", "", "BP GS", "University of the Sunshine Coast", "Maroochydore DC Qld", "University of the Sunshine Coast", "", "Maroochydore DC Qld", "", ""]]
  out "PP":string[][](table)=[["6025", "", "PP", "King Edward Memorial", "Perth", "Gemma McLeod", "mcleod.gemma1@gmail.com", "Perth", "", ""], ["6088", "", "PP", "Univ. of Sydney", "Penrith", "Ralph Nanan", "ralph.nanan@sydney.edu.au", "Penrith", "", ""], ["6021", "", "PP", "University of Queensland Centre for Clinical Research", "Herston", "Barbara Lingwood", "b.lingwood@uq.edu.au", "Herston", "", ""], ["6023", "", "PP", "University of Queensland Centre for Clinical Research", "Herston", "Barbara Lingwood", "b.lingwood@uq.edu.au", "Herston", "", ""], ["6082", "", "PP", "Massey Univ.", "Palmerston North", "Jane Coad", "CoadJ.Coad@massey.ac.nz", "Palmerston North", "", ""], ["6044", "", "PP", "Royal Prince Alfred Hospital", "Camperdown", "Emily Bek", "emily.bek@sydney.edu.au", "Camperdown", "", ""]]
  in  "Save Button":bool
  in  "Delete Item":bool
  in  "Send Follow Up":bool
  in  "Search Item":bool
  in  "Edit Item":bool
  in  "New Item":bool
  out "Item Selected (S/N):":string
  out "statuBar":string
  in  "Stop Button":bool
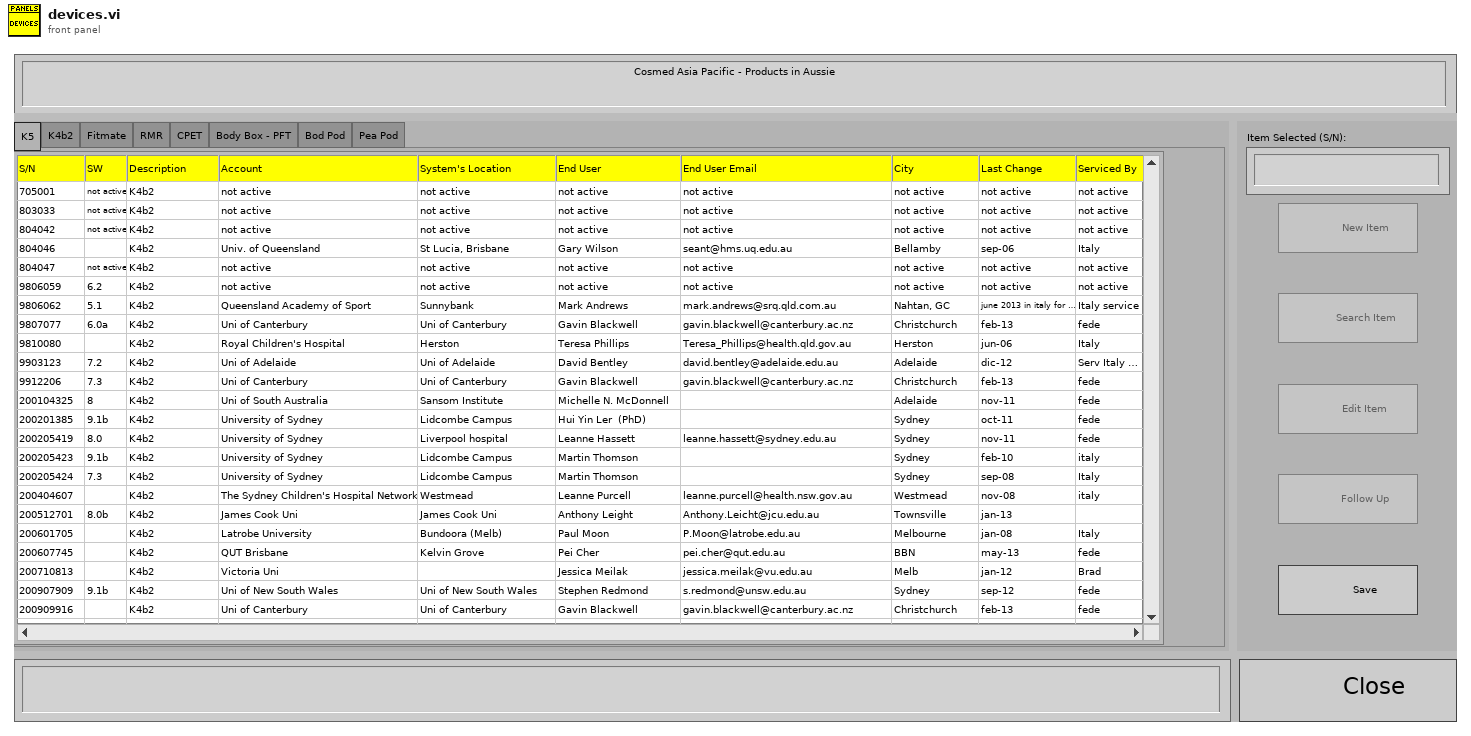
[diagram p1: front panel]
types:
  T1 = enum32{"K5", "K4b2", "Fitmate", "RMR", "CPET", "Body Box - PFT", "Bod Pod", "Pea Pod"}
  T2 = typedef "Project Panels.lvclass/state.ctl" = enum16{"initiate", "waitEvent", "newItem", "searchItem", "editItem", "sendFollowUp", "deleteItem", "save", "stop"}
  T3 = typedef "LVRowAndColumnUnsignedTypeDef.ctl" = cluster{"Row":u32, "Column":u32}
  T4 = enum8{"Enabled", "Disabled", "Disabled and Grayed Out"}
  T5 = typedef "Devices Controller.lvclass/deviceType.ctl" = enum16{"k5", "k4b2", "fitmate", "cpet", "rmr", "bodyBoxPft", "bp", "pp"}
  T6 = typedef "LVRowAndColumnTypeDef.ctl" = cluster{"Row":i32, "Column":i32}
  T7 = typedef "excelFile.lvclass/fileType.ctl" = enum16{"devices", "items", "partsTracking", "TSR"}
  T8 = typedef "Project Panels.lvclass/ObjectAttributesRef.ctl" = refnum<data-value>
  T9 = typedef "Project Panels.lvclass/ObjectAttributes.ctl" = cluster{"MyAttribute":dbl, "device_controller_ref":refnum<class "Devices Controller.lvclass">, "file_controller_ref":refnum<class "File Controller.lvclass">, "item_controller_ref":refnum<class "Items Controller.lvclass">, "item_tables":cluster{"checkIN":string[][], "checkOUT":string[][], "storage":string[][]}, "quickbook_table":cluster{"notes":string[][]}, "notification_controller_ref":refnum<class "Notification Controller.lvclass">, "partstracking_controller_ref":refnum<class "PartsTracking Controller.lvclass">, "product_tables":cluster{"k4b2":string[][], "fitmate":string[][], "RMR":string[][], "CPET":string[][], "BP":string[][], "PP":string[][], "k5":string[][], "bb-pft":string[][]}, "rowsColour":u32[], "low_resolution?":bool, "run_python?":bool}
  T10 = cluster{"k4b2":string[][], "fitmate":string[][], "RMR":string[][], "CPET":string[][], "BP":string[][], "PP":string[][], "k5":string[][], "bb-pft":string[][]}
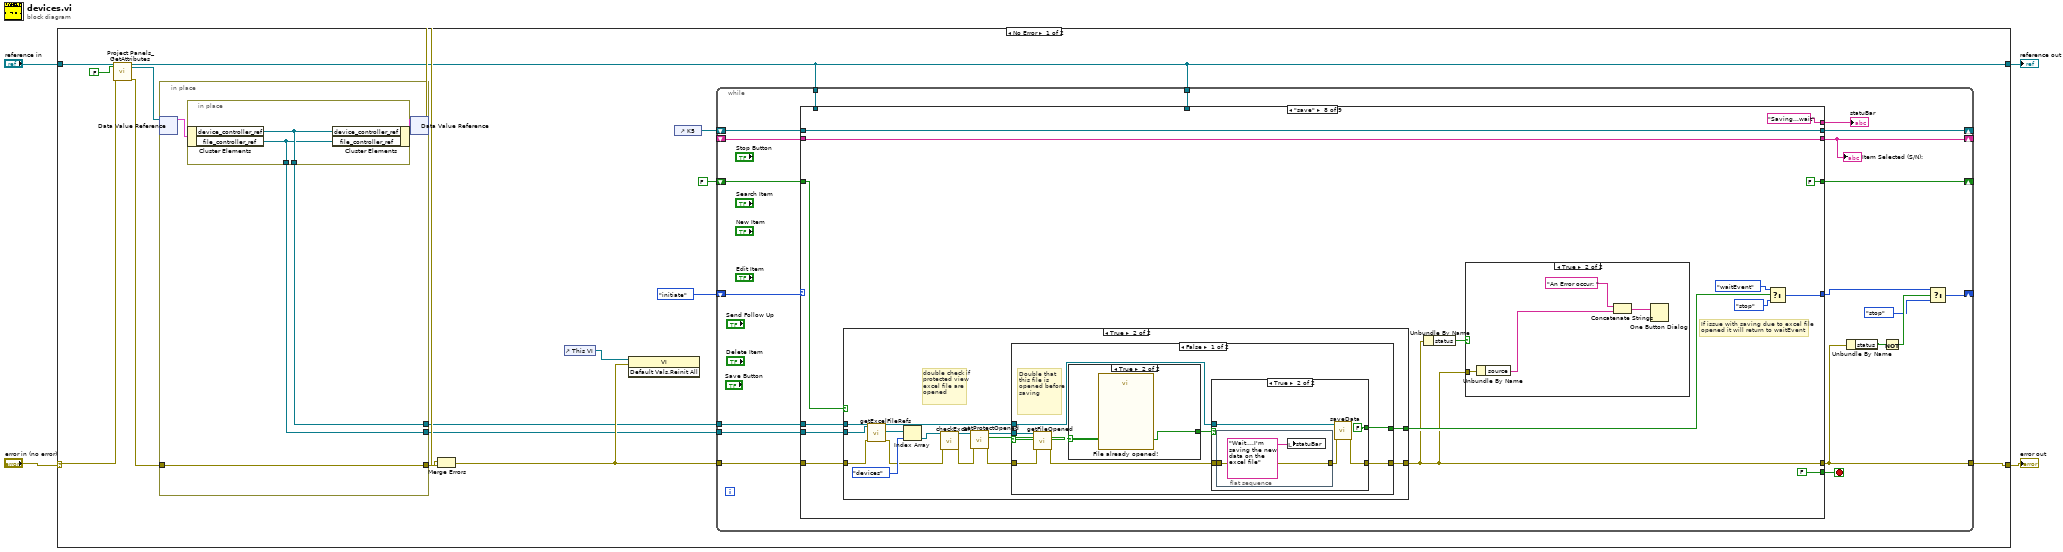
[diagram p0: block diagram]
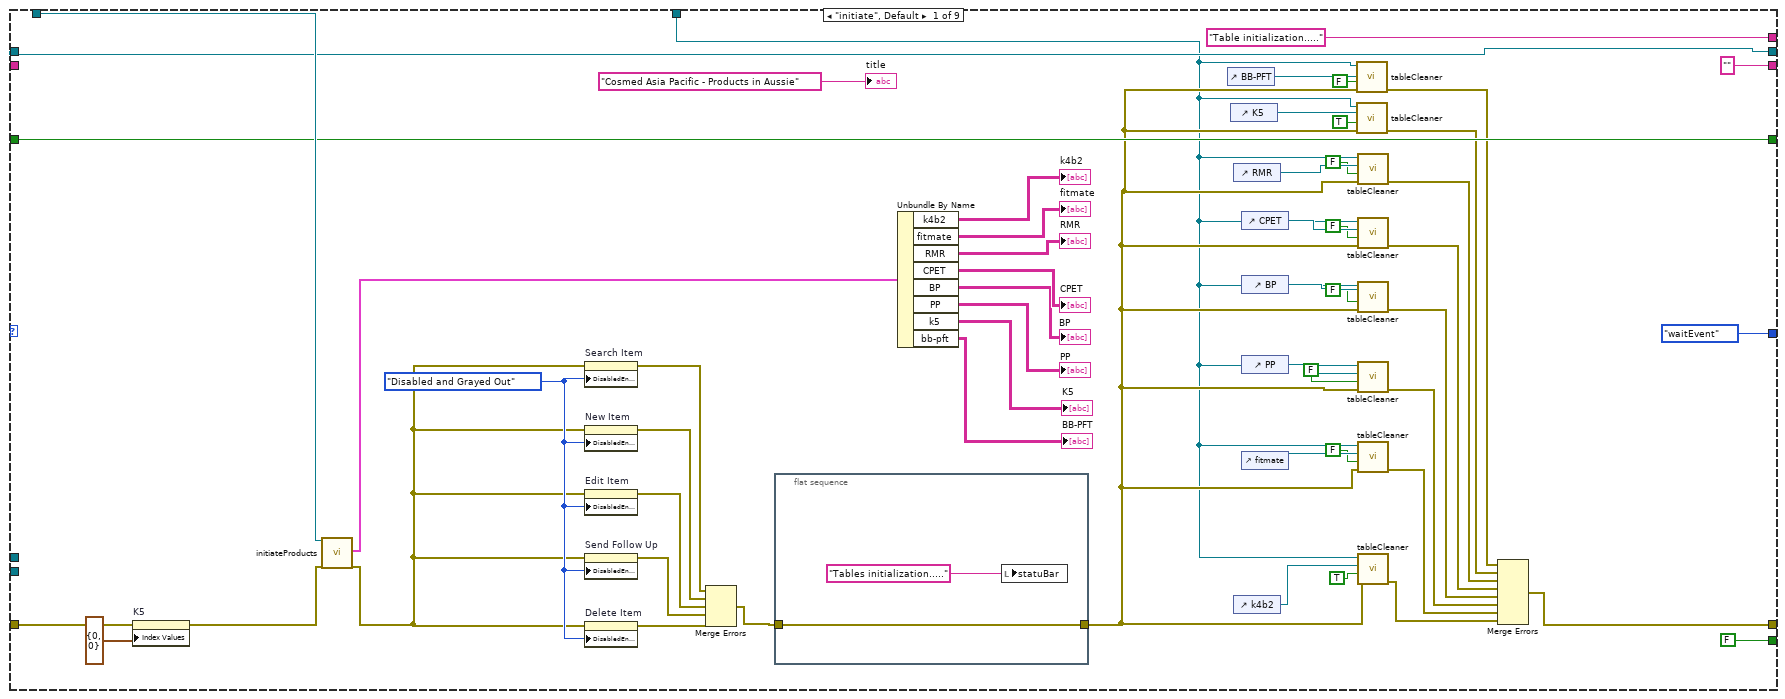
[diagram p2: hidden frame]
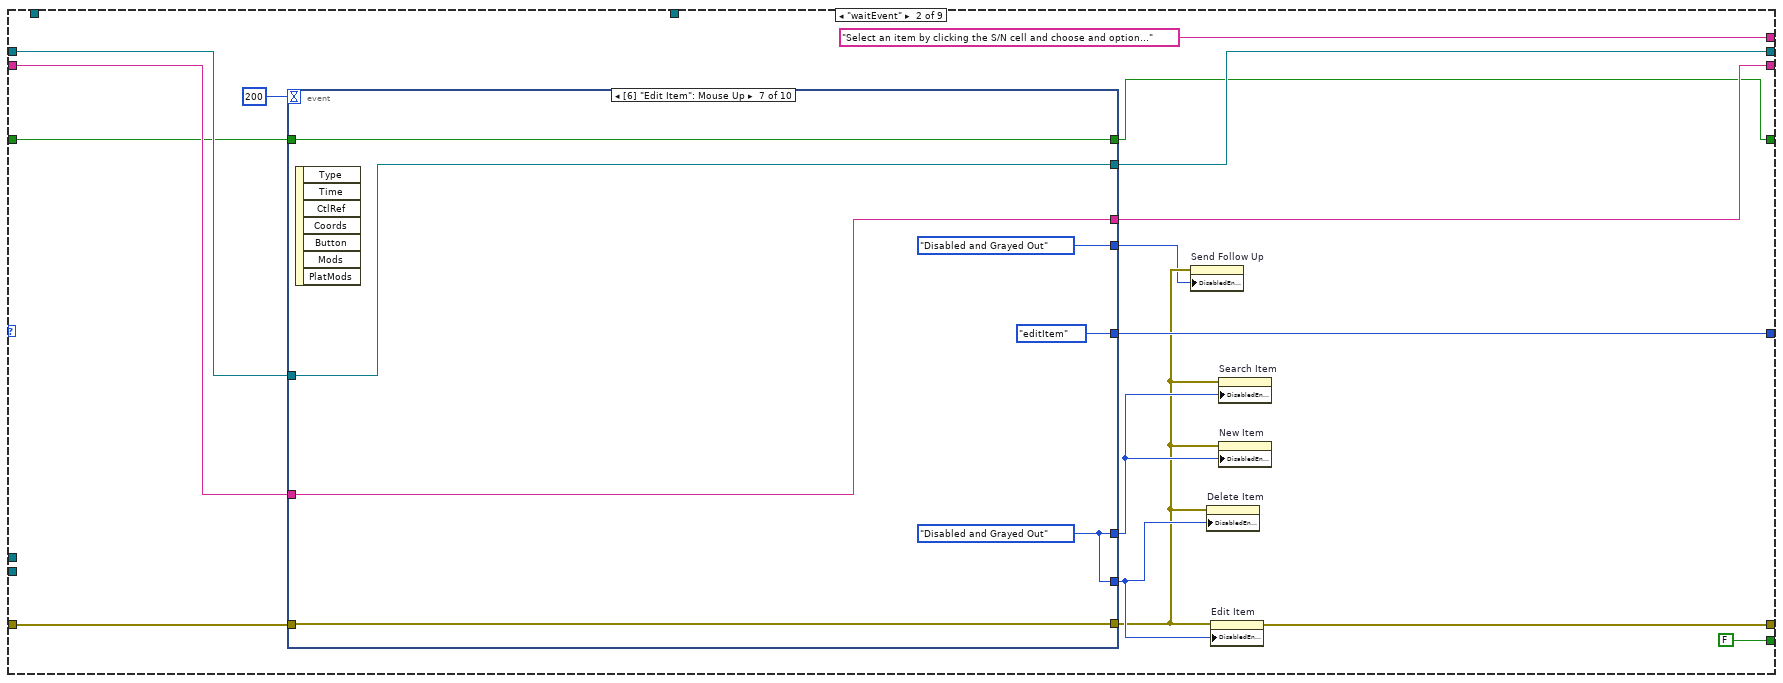
[diagram p3: hidden frame]
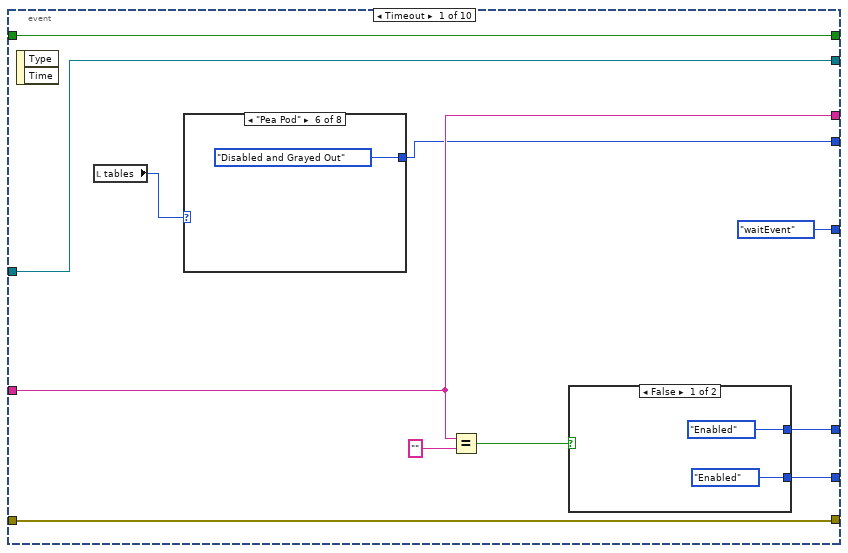
[diagram p4: hidden frame]
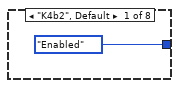
[diagram p5: hidden frame]
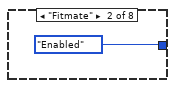
[diagram p6: hidden frame]
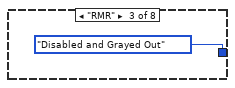
[diagram p7: hidden frame]
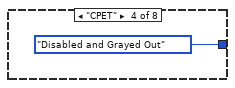
[diagram p8: hidden frame]
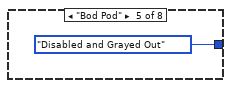
[diagram p9: hidden frame]
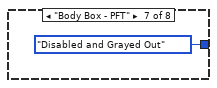
[diagram p10: hidden frame]
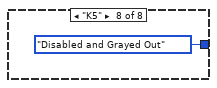
[diagram p11: hidden frame]
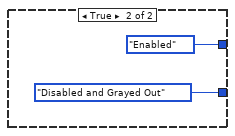
[diagram p12: hidden frame]
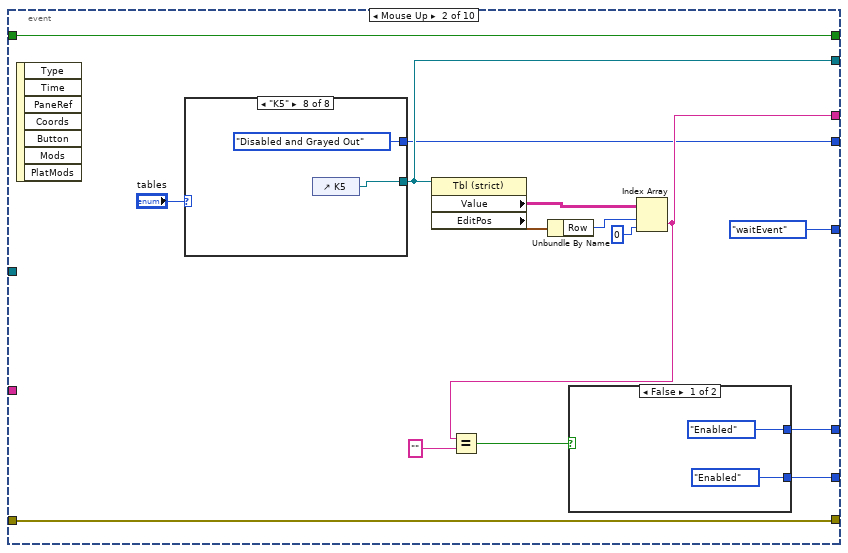
[diagram p13: hidden frame]
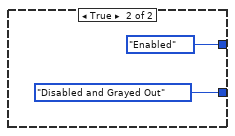
[diagram p14: hidden frame]
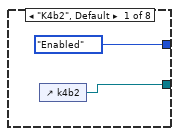
[diagram p15: hidden frame]
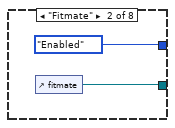
[diagram p16: hidden frame]
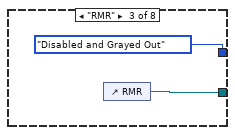
[diagram p17: hidden frame]
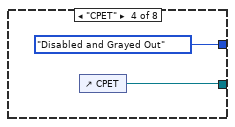
[diagram p18: hidden frame]
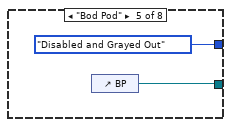
[diagram p19: hidden frame]
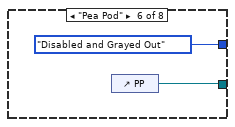
[diagram p20: hidden frame]
diagram:
  n1 = case shown="No Error" "error in (no error)" {
    selector: "error in (no error)" -> [w16 w451]
    tunnel: [w13 w451] -> w3
    tunnel: [w11 w450] -> w1
    tunnel: "reference in" -> [w18 w450]
    frame No Error {
      n2 = call "Project Panels_GetAttributes.vi"("reference in"=w18, "return data? (T)"=FALSE, "error in (no error)"=w16) -> ("reference out"=w11:refnum<class "Project Panels.lvclass">, "attributes ref"=w14:T8, "error out"=w15:errorcluster)  [unwired: 13 in, 1 out]
      n3 = in-place {
        in-place-border: w15 -> [w445]
        in-place-border: [w445] -> w19
        in-place-border: [w444] -> w6
        in-place-border: [w443] -> w5
        n4 = in-place-dvr #1(w14) -> (w446:T9)  [unwired: 1 out]
        n5 = in-place {
          in-place-border: [w449] -> w444
          in-place-border: [w448] -> w443
          n6 = in-place-cluster #2(w446) -> ("device_controller_ref"=w449:refnum<class "Devices Controller.lvclass">, "file_controller_ref"=w448:refnum<class "File Controller.lvclass">)
          n7 = in-place-cluster #2("device_controller_ref"=w449, "file_controller_ref"=w448) -> (w447:T9)
        }
        n8 = in-place-dvr #1(w447) -> (w20:errorcluster)  [unwired: 1 out]
      }
      n9 = Merge Errors(w19, w20) -> (w8:errorcluster)
      n10 = control-ref of="This VI"() -> (w9:refnum<vi>)
      n11 = invoke class="VI" method="Default Vals.Reinit All"(reference=w9, error in=w8) -> ()  [unwired: 1 in, 3 out]
      n12 = control-ref of="K5"() -> (w10:refnum<vi>)
      n13 = while {
        tunnel: w11 -> [w40]
        tunnel: w8 -> [w39]
        tunnel: [w37] -> w13
        shift-right: [w34] -> _
        shift-left: state."initiate" ("state") -> [w38]
        shift-right: [w29] -> _
        shift-left: _ -> [w28]
        shift-right: [w27] -> _
        shift-left: w10 -> [w26]
        tunnel: w11 -> [w25]
        shift-right: [w24] -> _
        shift-left: FALSE ("saved?") -> [w23]
        tunnel: w6 -> [w22]
        tunnel: w5 -> [w21]
        stop <- w31 stop-if-true
        n14 = case shown="\"save\"" w38 {
          tunnel: w40 -> [w47 _ w245 w269 w298 w316 w358 _ _]
          tunnel: w39 -> [w43 w112 w247 w268 w296 w319 w357 w371 w434]
          tunnel: [w44 w103 w243 w267 w281 w311 w359 w373 w434] -> w37
          tunnel: [state."waitEvent" ("state") w110 w240 w264 w280 w314 w351 w377 w428] -> w35
          tunnel: [FALSE FALSE FALSE FALSE FALSE FALSE FALSE FALSE TRUE] -> w31
          tunnel: ["Table initialization....." ("title") "Select an item by clicking the S/N cell and choose and option..." ("title") "New Item option selected...." ("title") "Search Item option selected..." ("title") "Edit Item option selected..." ("title") "Send Follow Up option selected" ("title") "Delete Item option selected..." ("title") "Saving...wait" ("title") w432] -> w30
          tunnel: ["" w102 "" "" w289 w315 w354 w383 ""] -> w29
          tunnel: w28 -> [_ w108 _ _ w289 w315 w354 w383 _]
          tunnel: [w57 w101 w248 w270 w293 w318 w355 w382 w438] -> w27
          tunnel: w26 -> [w57 w104 w248 w270 w293 w318 w355 w382 w438]
          tunnel: w25 -> [w58 _ _ _ _ _ _ _ _]
          tunnel: [w55 w98 w239 w262 w276 w313 w349 FALSE ("saved?") FALSE ("saved?")] -> w24
          tunnel: w23 -> [w55 w99 w236 w260 w274 w313 w347 w381 w430]
          tunnel: w22 -> [_ _ _ _ _ _ _ w380 _]
          tunnel: w21 -> [_ _ _ _ _ _ _ w370 _]
          frame "initiate", Default {
            w60 = T4."Disabled and Grayed Out" ("Disabled")
            n15 = property on="K5" class="Tbl (strict)"(error in=w43, "Index Values"=T3 {"Row"=0, "Column"=0}) -> (error out=w42:errorcluster)  [unwired: 1 in, 1 out]
            n16 = call "initiateProducts.vi"("reference in"=w58, "error in (no error)"=w42) -> ("tables"=w56:T10, "error out"=w59:errorcluster)  [unwired: 15 in, 1 out]
            n17 = property on="Search Item" class="Bool"(error in=w59, "DisabledEnum"=w60) -> (error out=w61:errorcluster)  [unwired: 1 in, 1 out]
            n18 = property on="New Item" class="Bool"(error in=w59, "DisabledEnum"=w60) -> (error out=w62:errorcluster)  [unwired: 1 in, 1 out]
            n19 = property on="Edit Item" class="Bool"(error in=w59, "DisabledEnum"=w60) -> (error out=w63:errorcluster)  [unwired: 1 in, 1 out]
            n20 = property on="Send Follow Up" class="Bool"(error in=w59, "DisabledEnum"=w60) -> (error out=w64:errorcluster)  [unwired: 1 in, 1 out]
            n21 = property on="Delete Item" class="Bool"(error in=w59, "DisabledEnum"=w60) -> (error out=w65:errorcluster)  [unwired: 1 in, 1 out]
            n22 = Merge Errors(w61, w62, w63, w64, w65) -> (w66:errorcluster)
            n23 = flat-sequence {
              tunnel: w66 -> [w97]
              tunnel: [w97] -> w52
              frame #0 {
                n24 = local write "statuBar"("Tables initialization....." ("title")) -> ()
              }
            }
            n25 = Unbundle By Name(w56) -> ("k4b2"=→"k4b2":string[][], "fitmate"=→"fitmate":string[][], "RMR"=→"RMR":string[][], "CPET"=→"CPET":string[][], "BP"=→"BP":string[][], "PP"=→"PP":string[][], "k5"=→"K5":string[][], "bb-pft"=→"BB-PFT":string[][])
            n26 = control-ref of="BB-PFT"() -> (w46:refnum<vi>)
            n27 = control-ref of="K5"() -> (w49:refnum<vi>)
            n28 = control-ref of="RMR"() -> (w87:refnum<vi>)
            n29 = control-ref of="k4b2"() -> (w89:refnum<vi>)
            n30 = control-ref of="CPET"() -> (w86:refnum<vi>)
            n31 = control-ref of="BP"() -> (w85:refnum<vi>)
            n32 = control-ref of="PP"() -> (w84:refnum<vi>)
            n33 = control-ref of="fitmate"() -> (w88:refnum<vi>)
            n34 = call "tableCleaner.vi"("error in (no error)"=w52, "K4b2orK5?"=FALSE, "Table in"=w46, "reference in"=w47) -> ("error out"=w50:errorcluster)  [unwired: 6 in, 1 out]
            n35 = call "tableCleaner.vi"("error in (no error)"=w52, "K4b2orK5?"=TRUE, "Table in"=w49, "reference in"=w47) -> ("error out"=w51:errorcluster)  [unwired: 6 in, 1 out]
            n36 = call "tableCleaner.vi"("error in (no error)"=w52, "K4b2orK5?"=FALSE ("K4b2?"), "Table in"=w87, "reference in"=w47) -> ("error out"=w77:errorcluster)  [unwired: 6 in, 1 out]
            n37 = call "tableCleaner.vi"("error in (no error)"=w52, "K4b2orK5?"=FALSE ("K4b2?"), "Table in"=w86, "reference in"=w47) -> ("error out"=w76:errorcluster)  [unwired: 6 in, 1 out]
            n38 = call "tableCleaner.vi"("error in (no error)"=w52, "K4b2orK5?"=FALSE ("K4b2?"), "Table in"=w85, "reference in"=w47) -> ("error out"=w75:errorcluster)  [unwired: 6 in, 1 out]
            n39 = call "tableCleaner.vi"("error in (no error)"=w52, "K4b2orK5?"=FALSE ("K4b2?"), "Table in"=w84, "reference in"=w47) -> ("error out"=w74:errorcluster)  [unwired: 6 in, 1 out]
            n40 = call "tableCleaner.vi"("error in (no error)"=w52, "K4b2orK5?"=FALSE ("K4b2?"), "Table in"=w88, "reference in"=w47) -> ("error out"=w73:errorcluster)  [unwired: 6 in, 1 out]
            n41 = call "tableCleaner.vi"("error in (no error)"=w52, "K4b2orK5?"=TRUE ("K4b2?"), "Table in"=w89, "reference in"=w47) -> ("error out"=w72:errorcluster)  [unwired: 6 in, 1 out]
            n42 = Merge Errors(w50, w51, w77, w76, w75, w74, w73, w72) -> (w44:errorcluster)
            "title" <- "Cosmed Asia Pacific - Products in Aussie" ("title")
          }
          frame "waitEvent" {
            n43 = event shown="[6] \"Edit Item\": Mouse Up" {
              selector: _ -> [_ _ _ _ _ _ _ _ _ _]
              dyn-events: _ -> [_ _ _ _ _ _ _ _ _ _]
              timeout: 200 -> [_ _ _ _ _ _ _ _ _ _]
              tunnel: w112 -> [w124 w151 w177 w184 w199 w205 w211 w218 w226 w232]
              tunnel: [w124 w151 w177 w184 w199 w205 w211 w218 w226 w232] -> w105
              tunnel: [state."waitEvent" ("state") state."waitEvent" ("state") state."newItem" ("state") state."searchItem" ("state") w187 state."stop" ("state") state."editItem" ("state") state."save" ("state") state."sendFollowUp" ("state") state."deleteItem" ("state")] -> w110
              tunnel: [w122 w139 w176 w183 w198 w204 w212 w219 w225 w233] -> w107
              tunnel: w108 -> [w117 _ w174 w181 w196 _ w209 w216 w223 w230]
              tunnel: [w119 w140 w176 w183 w198 w204 w212 w219 w225 w233] -> w106
              tunnel: w104 -> [w118 _ w175 w182 w197 w202 w210 w217 w224 w231]
              tunnel: [w117 w141 w174 w181 w196 "" w209 w216 w223 w230] -> w102
              tunnel: [w118 w145 w175 w182 w197 w202 w210 w217 w224 w231] -> w101
              tunnel: [w115 w138 T4."Disabled and Grayed Out" ("Disabled") T4."Disabled and Grayed Out" ("Disabled") T4."Disabled and Grayed Out" ("Disabled") T4."Disabled and Grayed Out" ("Disabled") T4."Disabled and Grayed Out" ("Disabled") T4."Disabled and Grayed Out" ("Disabled") T4."Disabled and Grayed Out" ("Disabled") T4."Disabled and Grayed Out" ("Disabled")] -> w100
              tunnel: w99 -> [w114 w137 w172 w179 w186 w200 w207 _ w221 w228]
              tunnel: [w114 w137 w172 w179 w186 w200 w207 TRUE ("saved?") w221 w228] -> w98
              event Timeout {
                n44 = event-data() -> ()  [unwired: 1 in, 2 out]
                n45 = local read "tables"() -> (w116:T1)
                n46 = case shown="\"Pea Pod\"" w116 {
                  tunnel: [T4."Enabled" ("Disabled") T4."Enabled" ("Disabled") T4."Disabled and Grayed Out" ("Disabled") T4."Disabled and Grayed Out" ("Disabled") T4."Disabled and Grayed Out" ("Disabled") T4."Disabled and Grayed Out" ("Disabled") T4."Disabled and Grayed Out" ("Disabled") T4."Disabled and Grayed Out" ("Disabled")] -> w115
                  frame "K4b2", Default {
                  }
                  frame "Fitmate" {
                  }
                  frame "RMR" {
                  }
                  frame "CPET" {
                  }
                  frame "Bod Pod" {
                  }
                  frame "Pea Pod" {
                  }
                  frame "Body Box - PFT" {
                  }
                  frame "K5" {
                  }
                }
                n47 = Equal?(x=w117, y="") -> (x = y?=w121:bool)
                n48 = case shown="False" w121 {
                  tunnel: [T4."Enabled" ("Disabled") T4."Disabled and Grayed Out" ("Disabled")] -> w122
                  tunnel: [T4."Enabled" ("Disabled") T4."Enabled" ("Disabled")] -> w119
                  frame False {
                  }
                  frame True {
                  }
                }
              }
              event Mouse Up {
                n49 = event-data() -> ()  [unwired: 1 in, 7 out]
                n50 = case shown="\"K5\"" "tables" {
                  tunnel: [w157 w159 w161 w163 w165 w167 w168 w170] -> w145
                  tunnel: [T4."Enabled" ("Disabled") T4."Enabled" ("Disabled") T4."Disabled and Grayed Out" ("Disabled") T4."Disabled and Grayed Out" ("Disabled") T4."Disabled and Grayed Out" ("Disabled") T4."Disabled and Grayed Out" ("Disabled") T4."Disabled and Grayed Out" ("Disabled") T4."Disabled and Grayed Out" ("Disabled")] -> w138
                  frame "K4b2", Default {
                    n51 = control-ref of="k4b2"() -> (w157:refnum<vi>)
                  }
                  frame "Fitmate" {
                    n52 = control-ref of="fitmate"() -> (w159:refnum<vi>)
                  }
                  frame "RMR" {
                    n53 = control-ref of="RMR"() -> (w161:refnum<vi>)
                  }
                  frame "CPET" {
                    n54 = control-ref of="CPET"() -> (w163:refnum<vi>)
                  }
                  frame "Bod Pod" {
                    n55 = control-ref of="BP"() -> (w165:refnum<vi>)
                  }
                  frame "Pea Pod" {
                    n56 = control-ref of="PP"() -> (w167:refnum<vi>)
                  }
                  frame "Body Box - PFT" {
                    n57 = control-ref of="BB-PFT"() -> (w168:refnum<vi>)
                  }
                  frame "K5" {
                    n58 = control-ref of="K5"() -> (w170:refnum<vi>)
                  }
                }
                n59 = property on="Property Node" class="Tbl (strict)"(reference=w145) -> ("Value"=w149:string[][], "EditPos"=w150:T6)  [unwired: 1 in, 2 out]
                n60 = Unbundle By Name(w150) -> ("Row"=w147:i32)
                n61 = Index Array(array=w149, index (row)=w147, index (col)=0 ("disabled index (col)")) -> (element=w141:string)
                n62 = Equal?(x=w141, y="") -> (x = y?=w143:bool)
                n63 = case shown="False" w143 {
                  tunnel: [T4."Enabled" ("Disabled") T4."Disabled and Grayed Out" ("Disabled")] -> w139
                  tunnel: [T4."Enabled" ("Disabled") T4."Enabled" ("Disabled")] -> w140
                  frame False {
                  }
                  frame True {
                  }
                }
              }
              event "New Item": Mouse Up {
                w176 = T4."Disabled and Grayed Out" ("Disabled")
                n64 = event-data() -> ()  [unwired: 1 in, 7 out]
              }
              event "Search Item": Mouse Up {
                w183 = T4."Disabled and Grayed Out" ("Disabled")
                n65 = event-data() -> ()  [unwired: 1 in, 7 out]
              }
              event Key Down? {
                w198 = T4."Disabled and Grayed Out" ("Disabled")
                n66 = event-data() -> ("Char"=w190:i16)  [unwired: 1 in, 9 out]
                n67 = To Unsigned Byte Integer(number=w190) -> (unsigned 8bit integer=w194:u8)
                n68 = Type Cast(x=w194) -> (*(type *) &x=w193:string)  [unwired: 1 in]
                n69 = Equal?(x=w193, y="f") -> (x = y?=w191:bool)
                n70 = Select(t=state."searchItem" ("state"), s=w191, f=state."waitEvent" ("state")) -> (s? t:f=w187:T2)
                n71 = event-data() -> ()  [unwired: 2 in, 1 out]
              }
              event "Stop Button": Mouse Up {
                w204 = T4."Disabled and Grayed Out" ("Disabled")
                n72 = event-data() -> ()  [unwired: 1 in, 7 out]
              }
              event "Edit Item": Mouse Up {
                w212 = T4."Disabled and Grayed Out" ("Disabled")
                n73 = event-data() -> ()  [unwired: 1 in, 7 out]
              }
              event "Save Button": Mouse Up {
                w219 = T4."Disabled and Grayed Out" ("Disabled")
                n74 = event-data() -> ()  [unwired: 1 in, 7 out]
              }
              event "Send Follow Up": Mouse Up {
                w225 = T4."Disabled and Grayed Out" ("Disabled")
                n75 = event-data() -> ()  [unwired: 1 in, 7 out]
              }
              event "Delete Item": Mouse Up {
                w233 = T4."Disabled and Grayed Out" ("Disabled")
                n76 = event-data() -> ()  [unwired: 1 in, 7 out]
              }
            }
            n77 = property on="Send Follow Up" class="Bool"(error in=w105, "DisabledEnum"=w100) -> ()  [unwired: 1 in, 2 out]
            n78 = property on="Delete Item" class="Bool"(error in=w105, "DisabledEnum"=w107) -> ()  [unwired: 1 in, 2 out]
            n79 = property on="Edit Item" class="Bool"(error in=w105, "DisabledEnum"=w107) -> (error out=w103:errorcluster)  [unwired: 1 in, 1 out]
            n80 = property on="Search Item" class="Bool"(error in=w105, "DisabledEnum"=w106) -> ()  [unwired: 1 in, 2 out]
            n81 = property on="New Item" class="Bool"(error in=w105, "DisabledEnum"=w106) -> ()  [unwired: 1 in, 2 out]
          }
          frame "newItem" {
            n82 = property class="Tbl (strict)"(reference=w248, error in=w247) -> (error out=w244:errorcluster, "Label.Text"=w246:string)  [unwired: 1 out]
            n83 = case shown="\"K5\"" w246 {
              tunnel: [deviceType."rmr" ("deviceType") deviceType."bodyBoxPft" ("deviceType") deviceType."fitmate" ("deviceType") deviceType."bp" ("deviceType") deviceType."pp" ("deviceType") deviceType."cpet" ("deviceType") deviceType."k4b2" ("deviceType") deviceType."k5" ("deviceType")] -> w235
              frame "RMR", Default {
              }
              frame "BB-PFT" {
              }
              frame "fitmate" {
              }
              frame "BP" {
              }
              frame "PP" {
              }
              frame "CPET" {
              }
              frame "k4b2" {
              }
              frame "K5" {
              }
            }
            n84 = call "newDevice.vi"("error in (no error)"=w244, "Device Type"=w235, "reference in"=w245) -> ("error out"=w243:errorcluster, "saved?"=w237:bool)  [unwired: 6 in, 1 out]
            n85 = Select(t=TRUE ("saved?"), s=w236, f=w237) -> (s? t:f=w239:bool)
            n86 = Select(t=state."initiate" ("state"), s=w237, f=state."waitEvent" ("state")) -> (s? t:f=w240:T2)
          }
          frame "searchItem" {
            n87 = call "searchEditDevice.vi"("error in (no error)"=w268, "reference in"=w269) -> ("error out"=w267:errorcluster, "saved?"=w261:bool)  [unwired: 7 in, 1 out]
            n88 = Select(t=TRUE ("saved?"), s=w260, f=w261) -> (s? t:f=w262:bool)
            n89 = Select(t=state."initiate" ("state"), s=w261, f=state."waitEvent" ("state")) -> (s? t:f=w264:T2)
          }
          frame "editItem" {
            n90 = property class="Tbl (strict)"(reference=w293, error in=w296) -> (error out=w295:errorcluster, "Label.Text"=w297:string)  [unwired: 1 out]
            n91 = case shown="\"PP\"" w297 {
              tunnel: [deviceType."rmr" ("deviceType") deviceType."k5" ("deviceType") deviceType."bodyBoxPft" ("deviceType") deviceType."fitmate" ("deviceType") deviceType."bp" ("deviceType") deviceType."pp" ("deviceType") deviceType."cpet" ("deviceType") deviceType."k4b2" ("deviceType")] -> w294
              frame "RMR", Default {
              }
              frame "K5" {
              }
              frame "BB-PFT" {
              }
              frame "fitmate" {
              }
              frame "BP" {
              }
              frame "PP" {
              }
              frame "CPET" {
              }
              frame "k4b2" {
              }
            }
            n92 = call "editDevice.vi"("error in (no error)"=w295, "S/N IN"=w289, "Device Type In"=w294, "reference in"=w298) -> ("error out"=w282:errorcluster, "saved?"=w275:bool)  [unwired: 5 in, 1 out]
            n93 = property on="Property Node" class="Tbl (strict)"(reference=w293, error in=w282) -> (reference out=w288:refnum<vi>, error out=w283:errorcluster, "Value"=w292:string[][])
            n94 = Index Array(array=w292, index (col)=0 ("disabled index (col)")) -> (element=w290:string[])  [unwired: 1 in]
            n95 = Search 1D Array(1D array=w290, element=w289) -> (index of element=w285:i32)  [unwired: 1 in]
            n96 = Bundle By Name(cluster=T6 {"Row"=0, "Column"=0} ("Active Cell:Active Cell"), "Row"=w285, "Column"=0) -> (w286:T6)
            n97 = property on="Property Node" class="Tbl (strict)"(reference=w288, error in=w283, "Index Values"=w286) -> (error out=w281:errorcluster)  [unwired: 1 out]
            n98 = Select(t=TRUE ("saved?"), s=w274, f=w275) -> (s? t:f=w276:bool)
            n99 = Select(t=state."initiate" ("state"), s=w275, f=state."waitEvent" ("state")) -> (s? t:f=w280:T2)
          }
          frame "sendFollowUp" {
            n100 = property class="Tbl (strict)"(reference=w318, error in=w319) -> (error out=w317:errorcluster, "Label.Text"=w310:string)  [unwired: 1 out]
            n101 = case shown="\"K5\"" w310 {
              tunnel: [deviceType."rmr" ("deviceType") deviceType."k5" ("deviceType") deviceType."bodyBoxPft" ("deviceType") deviceType."fitmate" ("deviceType") deviceType."bodyBoxPft" ("deviceType") deviceType."bp" ("deviceType") deviceType."cpet" ("deviceType") deviceType."k4b2" ("deviceType")] -> w309
              frame "RMR", Default {
              }
              frame "K5" {
              }
              frame "BB-PFT" {
              }
              frame "fitmate" {
              }
              frame "BP" {
              }
              frame "PP" {
              }
              frame "CPET" {
              }
              frame "k4b2" {
              }
            }
            n102 = call "followUpDevice.vi"("error in (no error)"=w317, "S/N"=w315, "Device Type"=w309, "reference in"=w316) -> ("error out"=w312:errorcluster)  [unwired: 6 in, 1 out]
            n103 = case shown="No Error" w312 {
              selector: w312 -> [w330 w343]
              tunnel: [w331 state."waitEvent" ("state")] -> w314
              tunnel: [w330 w341] -> w311
              frame No Error {
                n104 = flat-sequence {
                  tunnel: [w334] -> w331
                  frame #0 {
                    n105 = Two Button Dialog(message="Do you want to update the Follow Up sent Date?", 1:"No" ("F button name (\"Cancel\")"), 2:"Yes" ("T button name (\"OK\")")) -> (T button?=w333:bool)
                    n106 = Select(t=state."editItem", s=w333, f=state."waitEvent" ("state")) -> (s? t:f=w334:T2)
                  }
                }
              }
              frame Error {
                n107 = call <vilib>:"Simple Error Handler.vi"("error in (no error)"=w343) -> ("source out"=w339:string, "error out"=w342:errorcluster)  [unwired: 4 in, 3 out]
                n108 = call <vilib>:"Clear Errors.vi"("error in (no error)"=w342) -> ("error out"=w341:errorcluster)  [unwired: 5 in, 1 out]
                n109 = One Button Dialog(message=w339, button name ("OK")="OK" ("T button name (\"OK\")")) -> ()  [unwired: 1 out]
              }
            }
          }
          frame "deleteItem" {
            n110 = property class="Tbl (strict)"(reference=w355, error in=w357) -> (error out=w356:errorcluster, "Label.Text"=w346:string)  [unwired: 1 out]
            n111 = case shown="\"K5\"" w346 {
              tunnel: [deviceType."rmr" ("deviceType") deviceType."k5" ("deviceType") deviceType."bodyBoxPft" ("deviceType") deviceType."fitmate" ("deviceType") deviceType."bodyBoxPft" ("deviceType") deviceType."bp" ("deviceType") deviceType."cpet" ("deviceType") deviceType."k4b2" ("deviceType")] -> w345
              frame "RMR", Default {
              }
              frame "K5" {
              }
              frame "BB-PFT" {
              }
              frame "fitmate" {
              }
              frame "BP" {
              }
              frame "PP" {
              }
              frame "CPET" {
              }
              frame "k4b2" {
              }
            }
            n112 = call "deleteDevice.vi"("error in (no error)"=w356, "S/N IN"=w354, "Device Type In"=w345, "reference in"=w358) -> ("error out"=w359:errorcluster, "saved?"=w348:bool)  [unwired: 5 in, 1 out]
            n113 = Select(t=TRUE ("saved?"), s=w347, f=w348) -> (s? t:f=w349:bool)
            n114 = Select(t=state."initiate" ("state"), s=w348, f=state."waitEvent" ("state")) -> (s? t:f=w351:T2)
          }
          frame "save" {
            # "If issue with saving due to excel file\nopened it will return to waitEvent"
            n115 = case shown="True" w381 {
              tunnel: w371 -> [w386 w395]
              tunnel: [w386 w400] -> w373
              tunnel: w380 -> [_ w399]
              tunnel: [TRUE ("saved?") w398] -> w376
              tunnel: w370 -> [_ w392]
              frame False {
              }
              frame True {
                # "double check if protected view excel file are opened"
                n116 = call "getExcelFileRefs.vi"("error in (no error)"=w395, "reference in"=w392) -> ("error out"=w389:errorcluster, "excelFile_refs"=w397:refnum<class "excelFile.lvclass">[])  [unwired: 7 in, 1 out]
                n117 = Index Array(array=w397, index=fileType."devices" ("fileType")) -> (element=w391:refnum<class "excelFile.lvclass">)
                n118 = call "checkExcel.vi"("reference in"=w391, "error in (no error)"=w389) -> ("reference out"=w390:refnum<class "excelFile.lvclass">, "error out"=w388:errorcluster)  [unwired: 16 in]
                n119 = call "getProtectOpened.vi"("error in (no error)"=w388, "reference in"=w390) -> ("error out"=w394:errorcluster, "excel_protected_opened?"=w393:bool, "reference out"=w387:refnum<class "excelFile.lvclass">)  [unwired: 7 in]
                n120 = case shown="False" w393 {
                  tunnel: [w408 w421] -> w400
                  tunnel: w394 -> [w405 w421]
                  tunnel: w399 -> [w407 _]
                  tunnel: [w401 TRUE ("protected_view?")] -> w398
                  tunnel: w387 -> [w403 _]
                  frame False {
                    # "Double that this file is opened before saving"
                    n121 = call "getFileOpened.vi"("error in (no error)"=w405, "reference in"=w403) -> ("error out"=w404:errorcluster, "file_already_opened?"=w406:bool)  [unwired: 7 in, 1 out]
                    n122 = case shown="True" w406 {
                      tunnel: [TRUE ("T button?") w419] -> w402
                      frame False {
                      }
                      frame True {
                        n123 = call "File already opened!"() -> ("Save"=w419:bool)  [unwired: 10 in, 1 out]
                      }
                    }
                    n124 = case shown="True" w402 {
                      tunnel: [w410 w415] -> w408
                      tunnel: w407 -> [_ w413]
                      tunnel: w404 -> [w410 w412]
                      tunnel: [TRUE ("protected_view?") FALSE ("protected_view?")] -> w401
                      frame False {
                      }
                      frame True {
                        n125 = flat-sequence {
                          tunnel: w412 -> [w416]
                          tunnel: [w416] -> w414
                          frame #0 {
                            n126 = local write "statuBar"("Wait....I'm saving the new data on the excel file" ("statuBar")) -> ()
                          }
                        }
                        n127 = call "saveData.vi"("error in (no error)"=w414, "reference in"=w413) -> ("error out"=w415:errorcluster)  [unwired: 8 in, 1 out]
                      }
                    }
                  }
                  frame True {
                    n128 = call "File opened in protected view!"() -> ()  [unwired: 10 in, 2 out]
                  }
                }
              }
            }
            n129 = Unbundle By Name(w373) -> ("status"=w372:bool)
            n130 = case shown="True" w372 {
              tunnel: w373 -> [_ w423]
              frame False {
              }
              frame True {
                n131 = Unbundle By Name(w423) -> ("source"=w422:string)
                n132 = Concatenate Strings("An Error occur: " ("message"), w422) -> (w425:string)
                n133 = One Button Dialog(message=w425) -> ()  [unwired: 1 in, 1 out]
              }
            }
            n134 = Select(t=state."waitEvent" ("state"), s=w376, f=state."stop" ("state")) -> (s? t:f=w377:T2)
          }
          frame "stop" {
            n135 = Unbundle By Name(w434) -> ("status"=w435:bool)
            n136 = Not(x=w435) -> (.not. x?=w433:bool)
            n137 = Select(t="Stoped from User" ("title"), s=w433, f="Stoped for an Error" ("title")) -> (s? t:f=w432:string)
            n138 = case shown="False" w430 {
              tunnel: [w441 FALSE ("Save")] -> w427
              frame False {
                n139 = call "Display Message to User"() -> ("Save"=w441:bool)  [unwired: 10 in, 1 out]
              }
              frame True {
              }
            }
            n140 = Select(t=state."save", s=w427, f=state."stop" ("state")) -> (s? t:f=w428:T2)
          }
        }
        "statuBar" <- w30
        "Item Selected (S/N):" <- w29
        n141 = Unbundle By Name(w37) -> ("status"=w36:bool)
        n142 = Not(x=w36) -> (.not. x?=w33:bool)
        n143 = Select(t=w35, s=w33, f=state."stop") -> (s? t:f=w34:T2)
      }
    }
    frame Error {
    }
  }
  "error out" <- w3
  "reference out" <- w1
